vi "Dead Zone (DBL Array).vi"(2 "end of dead zone":dbl format="%.2f", 3 "start of dead zone":dbl format="%.2f", 4 "Input Points":dbl[](array[numeric]) format="%.2f") -> (1 "Output Points":dbl[](array[numeric]) format="%.2f")   [LabVIEW 2020, in "NI_AdvCtrl_nonlinear.lvlib"]
doc: "LabVIEW no longer supports this VI. You can obtain similar functionality by installing the LabVIEW Simulation Module.\n\nRealizes a region of zero output, the so-called dead zone. The output is zero, if the inequalities start of dead zone < input < end of dead zone hold true."
uses:
  <vilib>/addons/control/advanced/NI_AdvCtrl_nonlinear.lvlib
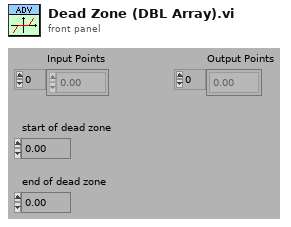
[diagram p1: front panel]
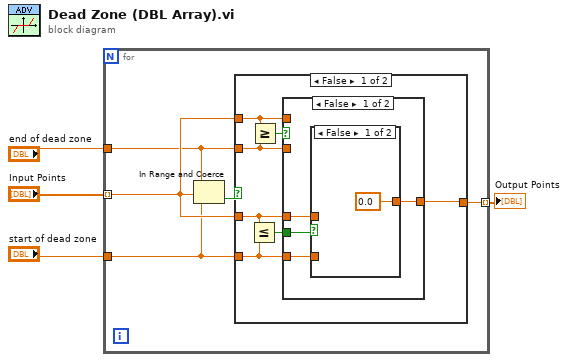
[diagram p0: block diagram]
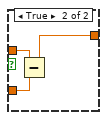
[diagram p2: hidden frame]
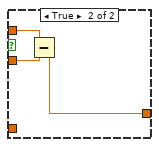
[diagram p3: hidden frame]
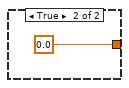
[diagram p4: hidden frame]
diagram:
  n1 = for {
    tunnel: "Input Points" -> [w8] mode=indexing
    tunnel: [w7] -> w3 mode=indexing
    tunnel: "end of dead zone" -> [w6]
    tunnel: "start of dead zone" -> [w5]
    n2 = In Range and Coerce(upper limit=w6, x=w8, lower limit=w5) -> (In Range?=w9:bool)  [unwired: 1 out]
    n3 = case shown="False" w9 {
      tunnel: [w13 0.0] -> w7
      tunnel: w6 -> [w14 _]
      tunnel: w8 -> [w15 _]
      tunnel: w8 -> [w11 _]
      tunnel: w5 -> [w10 _]
      frame False {
        n4 = Less Or Equal?(x=w11, y=w10) -> (x <= y?=w12:bool)
        n5 = Greater Or Equal?(x=w15, y=w14) -> (x >= y?=w16:bool)
        n6 = case shown="False" w16 {
          tunnel: w15 -> [_ w27]
          tunnel: w14 -> [_ w26]
          tunnel: [w17 w25] -> w13
          tunnel: w12 -> [w20 _]
          tunnel: w11 -> [w19 _]
          tunnel: w10 -> [w18 _]
          frame False {
            n7 = case shown="False" w20 {
              tunnel: w19 -> [_ w24]
              tunnel: w18 -> [_ w23]
              tunnel: [0.0 w22] -> w17
              frame False {
              }
              frame True {
                n8 = Subtract(x=w24, y=w23) -> (x-y=w22:dbl)
              }
            }
          }
          frame True {
            n9 = Subtract(x=w27, y=w26) -> (x-y=w25:dbl)
          }
        }
      }
      frame True {
      }
    }
  }
  "Output Points" <- w3
